vi "Main.vi"   [LabVIEW 2019]
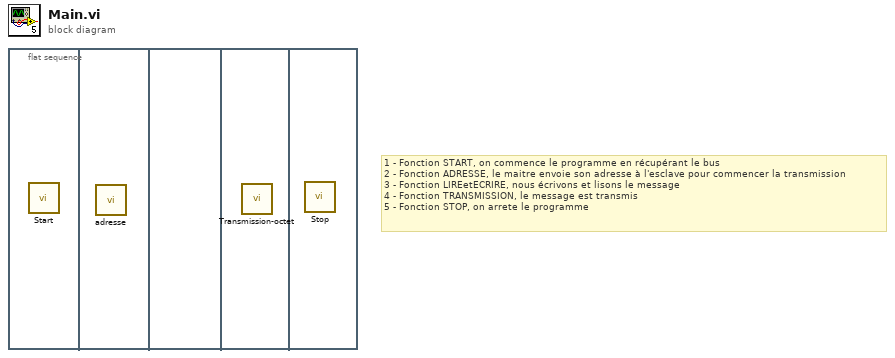
[diagram p0: block diagram]
diagram:
  # "1 - Fonction START, on commence le programme en récupérant le bus\n2 - Fonction ADRESSE, le maitre envoie son adresse à l'esclave pour commencer la transmission\n3 - Fonction LIREetECRIRE, nous écrivons et lisons le message\n4 - Fonction TRANSMISSION, le message est transmis\n5 - Fonction STOP, on arrete le programme"
  n1 = flat-sequence {
    frame #0 {
      n2 = call "Start.vi"() -> ()  [unwired: 12 in]
    }
    frame #1 {
      n3 = call "adresse.vi"() -> ()  [unwired: 12 in]
    }
    frame #2 {
    }
    frame #3 {
      n4 = call "Transmission-octet.vi"() -> ()  [unwired: 12 in]
    }
    frame #4 {
      n5 = call "Stop.vi"() -> ()  [unwired: 12 in]
    }
  }
